vi "Robot To Field Centric.vi"(10 "Robot Centric Velocities":T1, 11 "IMU Value (offset)":dbl) -> (2 "Field Centric Velocities":T1, 3 "Wrapped IMU (radians)":dbl)   [LabVIEW 2023]
uses:
  Type Definitions/Data/Robot Velocities.ctl
  <vilib>/Analysis/coordinate.llb/Angle Units.ctl
  <vilib>/Analysis/coordinate.llb/Angle Range (Degree).ctl
  <vilib>/Analysis/coordinate.llb/Wrap Angle (scalar).vi
  <vilib>/Analysis/NI_AAL_Angle.lvlib
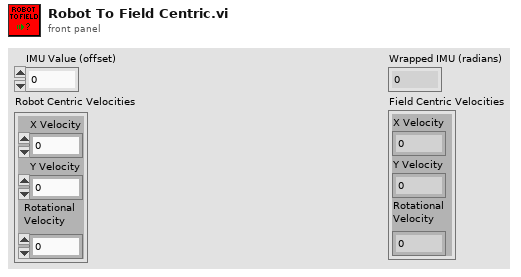
[diagram p1: front panel]
types:
  T1 = typedef "Robot Velocities.ctl" = cluster{"X Velocity":dbl, "Y Velocity":dbl, "Rotational \nVelocity":dbl}
  T2 = typedef "NI_AAL_Angle.lvlib/Angle Range (Degree).ctl" = u16
  T3 = typedef "NI_AAL_Angle.lvlib/Angle Units.ctl" = i32
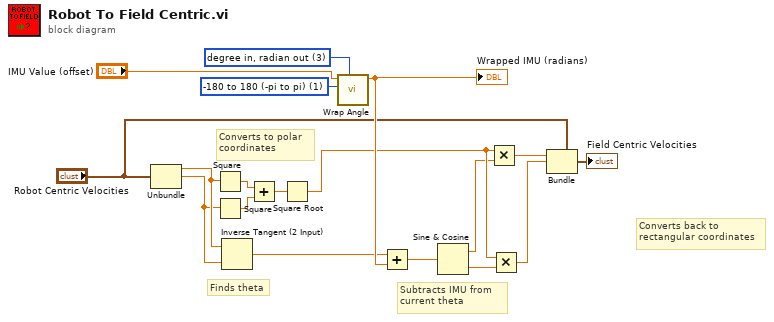
[diagram p0: block diagram]
diagram:
  w17 = T2 1 items=["none", "-180 to 180 (-pi to pi)", "0 to 360 (0 to 2pi)"] ("angle range")
  w18 = T3 3 items=["radian in, radian out", "radian in, degree out", "degree in, degree out", "degree in, radian out"] ("angle units")
  # "Converts back to \nrectangular coordinates"
  # "Subtracts IMU from \ncurrent theta"
  # "Finds theta"
  # "Converts to polar \ncoordinates"
  n1 = Unbundle("Robot Centric Velocities") -> ("X Velocity"=w5:dbl, "Y Velocity"=w4:dbl)  [unwired: 1 out]
  n2 = Square(x=w5) -> (x^2=w16:dbl)
  n3 = Square(x=w4) -> (x^2=w15:dbl)
  n4 = Inverse Tangent (2 Input)(1:w4, 2:w5) -> (0:w12:dbl)
  n5 = Add(x=w16, y=w15) -> (x+y=w14:dbl)
  n6 = Square Root(x=w14) -> (sqrt(x)=w11:dbl)
  n7 = call-poly <vilib>:"Wrap Angle.vi"("angle units"=w18, "angle range"=w17, "angle in"="IMU Value (offset)") -> ("angle out"=w13:dbl)  [unwired: 7 in, 1 out]
  "Wrapped IMU (radians)" <- w13
  n8 = Add(x=w12, y=w13) -> (x+y=w8:dbl)
  n9 = Sine & Cosine(0:w8) -> (1:w6:dbl, 2:w7:dbl)
  n10 = Multiply(x=w11, y=w6) -> (x*y=w10:dbl)
  n11 = Multiply(x=w11, y=w7) -> (x*y=w9:dbl)
  n12 = Bundle(cluster="Robot Centric Velocities", "X Velocity"=w10, "Y Velocity"=w9) -> (→"Field Centric Velocities":T1)  [unwired: 1 in]
